vi "read_config_file.vi"(8 "error in (no error)":errorcluster, 10 "force load?":bool, 11 "GenericPlugin in":refnum<class "GenericComponent.lvclass">) -> (0 "error out":errorcluster, 3 "GenericPlugin out":refnum<class "GenericComponent.lvclass">)   [LabVIEW 2010, in "GenericComponent.lvclass"]
doc: "The dynamic dispatch version of this VI loads the config file from the config_files folder of the actual plug-in class. The name of the config file to be loaded is property of the plug-in object. If not explicitely set, a file config_files/config.xml is loaded by default."
uses:
  GenericComponent.lvclass
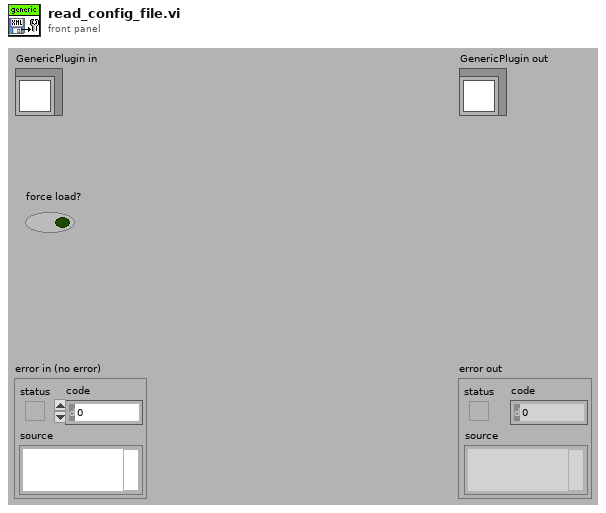
[diagram p1: front panel]
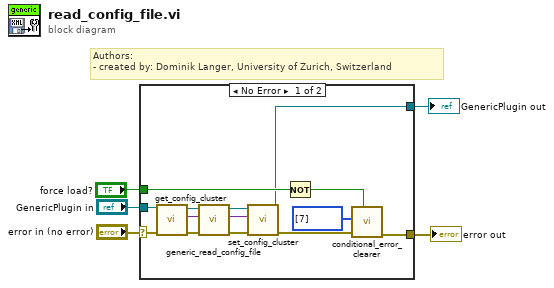
[diagram p0: block diagram]
diagram:
  # "Authors: \n- created by: Dominik Langer, University of Zurich, Switzerland"
  n1 = case shown="No Error" "error in (no error)" {
    selector: "error in (no error)" -> [w9 w21]
    tunnel: [w19 w21] -> w5
    tunnel: "force load?" -> [w18 _]
    tunnel: "GenericPlugin in" -> [w11 w20]
    tunnel: [w10 w20] -> w2
    frame No Error {
      n2 = call-dynamic "get_config_cluster.vi"("error in (no error)"=w9, "GenericComponent in"=w11) -> ("error out"=w17:errorcluster, "config cluster (variant)"=w16:variant, "GenericComponent out"=w15:refnum<class "GenericComponent.lvclass">)  [unwired: 7 in]
      n3 = call-dynamic "generic_read_config_file.vi"("error in (no error)"=w17, "config cluster variant in (data type)"=w16, "GenericPlugin in"=w15) -> ("error out"=w14:errorcluster, "config cluster variant out (populated"=w12:variant, "GenericPlugin out"=w13:refnum<class "GenericComponent.lvclass">)  [unwired: 6 out]
      n4 = call-dynamic "set_config_cluster.vi"("error in (no error)"=w14, "config cluster variant"=w12, "GenericComponent in"=w13) -> ("error out"=w7:errorcluster, "GenericComponent out"=w10:refnum<class "GenericComponent.lvclass">)  [unwired: 7 in]
      n5 = Not(x=w18) -> (.not. x?=w6:bool)
      n6 = call "conditional_error_clearer.vi"("clear?"=w6, "error in (no error)"=w7, "array of clearable error codes"=i32[] [7]) -> ("error out"=w19:errorcluster)  [unwired: 8 in]
    }
    frame Error {
    }
  }
  "error out" <- w5
  "GenericPlugin out" <- w2
